vi "Remove Group.vi"(8 "error in (no error)":errorcluster, 10 "ID":string, 11 "Configuration Session in":refnum<class "Configuration Session.lvclass">) -> (0 "error out":errorcluster, 3 "Configuration Session out":refnum<class "Configuration Session.lvclass">, 4 "exists?":bool)   [LabVIEW 2017, in "DSF Core.lvlib" / "Configuration Session.lvclass"]
doc: "Removes a section from the configuration data identified by <B>dsf refnum</B>."
uses:
  Configuration Session.lvclass
  Configuration Session.lvclass/Configuration Session.ctl
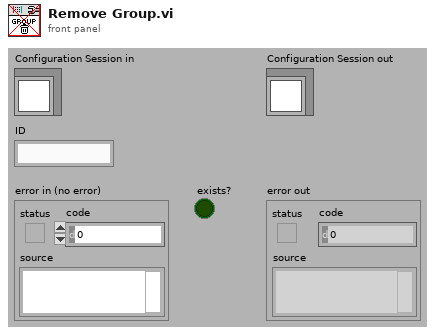
[diagram p1: front panel]
types:
  T1 = typedef "DSF Core.lvlib/Configuration Session.lvclass/DSF Config Data Ref.ctl" = refnum<data-value>
  T2 = typedef "DSF Core.lvlib/Configuration Session.lvclass/DSF Config Data.ctl" = cluster{"dsf configuration":T3, "path":path, "dirty":bool}
  T3 = typedef "DSF Core.lvlib/Configuration Session.lvclass/Internal DSF Configuration.ctl" = cluster{"dsfversion":T4, "version":T4, "plugins":T5[], "groups":T10[], "transfers":T12[], "channels":T14[], "settings":T16[], "framework configuration":T18}
  T4 = typedef "DSF Core.lvlib/DSF Version Info.ctl" = cluster{"major":u32, "minor":u32, "fix":u32, "build":string}
  T5 = typedef "DSF Core.lvlib/Configuration Session.lvclass/Internal DSF Plugin with ID.ctl" = cluster{"id":string, "values":T6}
  T6 = typedef "DSF Core.lvlib/Configuration Session.lvclass/Internal DSF Plugin Info.ctl" = cluster{"components":string[], "timing":T7, "group ids":string[], "settings id":string, "threads":T8[]}
  T7 = typedef "DSF Core.lvlib/DSF Timing Info.ctl" = cluster{"priority":u64, "decimation":u64, "offset":u64}
  T8 = typedef "DSF Core.lvlib/DSF Engine Plugin Thread Configuration.ctl" = cluster{"buffer converter settings":T9, "transceiver settings":T9, "custom settings":T9, "processor":i32, "priority offset":i16}
  T9 = typedef "DSF Core.lvlib/DSF Settings Info.ctl" = cluster{"key":string, "value":string}[]
  T10 = typedef "DSF Core.lvlib/Configuration Session.lvclass/Internal DSF Group with ID.ctl" = cluster{"id":string, "values":T11}
  T11 = typedef "DSF Core.lvlib/Configuration Session.lvclass/Internal DSF Group Info.ctl" = cluster{"direction":i32, "timing":T7, "transfer ids":string[], "settings id":string, "thread":i32, "timeout behavior":u8}
  T12 = typedef "DSF Core.lvlib/Configuration Session.lvclass/Internal DSF Transfer with ID.ctl" = cluster{"id":string, "values":T13}
  T13 = typedef "DSF Core.lvlib/Configuration Session.lvclass/Internal DSF Transfer Info.ctl" = cluster{"byte order":i32, "channel ids":string[], "settings id":string}
  T14 = typedef "DSF Core.lvlib/Configuration Session.lvclass/Internal DSF Channel with ID.ctl" = cluster{"id":string, "values":T15}
  T15 = typedef "DSF Core.lvlib/Configuration Session.lvclass/Internal DSF Channel Info.ctl" = cluster{"string buffer offset":u64, "string data type":i32, "engine data type":i32, "settings id":string, "units":string}
  T16 = typedef "DSF Core.lvlib/Configuration Session.lvclass/Internal DSF Settings with ID.ctl" = cluster{"id":string, "values":T17}
  T17 = typedef "DSF Core.lvlib/Configuration Session.lvclass/Internal DSF Settings Info.ctl" = cluster{"key":string, "value":string}[]
  T18 = typedef "DSF Core.lvlib/DSF Engine Framework Configuration.ctl" = cluster{"Plugins":T19[]}
  T19 = typedef "DSF Core.lvlib/DSF Engine Plugin Configuration.ctl" = cluster{"name":string, "components":string[], "cycle timing":T7, "threads":T8[], "Transfer Groups":T20[], "settings":T9}
  T20 = typedef "DSF Core.lvlib/DSF Engine Transfer Group Configuration.ctl" = cluster{"name":string, "direction":T21, "cycle timing":T7, "thread index":i32, "settings":T9, "Transfers":T22[], "timeout behavior":T26}
  T21 = typedef "DSF Core.lvlib/DSF Direction.ctl" = enum8{"Tx", "Rx"}
  T22 = typedef "DSF Core.lvlib/DSF Engine Transfer Configuration.ctl" = cluster{"name":string, "byte order":T23, "settings":T9, "channels":T24[]}
  T23 = typedef "DSF Core.lvlib/DSF Byte Order.ctl" = enum8{"big-endian", "little-endian"}
  T24 = typedef "DSF Core.lvlib/DSF Engine Channel Configuration.ctl" = cluster{"string offset":u64, "string data type":T25, "engine data type":T25, "name":string, "settings":T9, "units":string}
  T25 = typedef "DSF Core.lvlib/DSF Data Type.ctl" = enum8{"Bool", "SGL", "DBL", "I8", "I16", "I32", "I64", "U8", "U16", "U32", "U64"}
  T26 = typedef "DSF Core.lvlib/DSF Timeout Behavior.ctl" = enum8{"Increment Late Count", "Throw Error"}
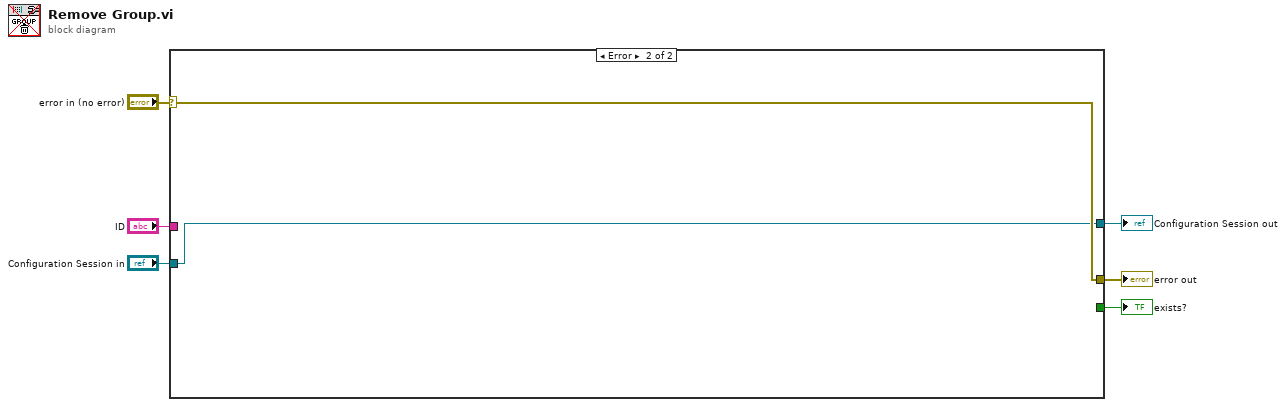
[diagram p0: block diagram]
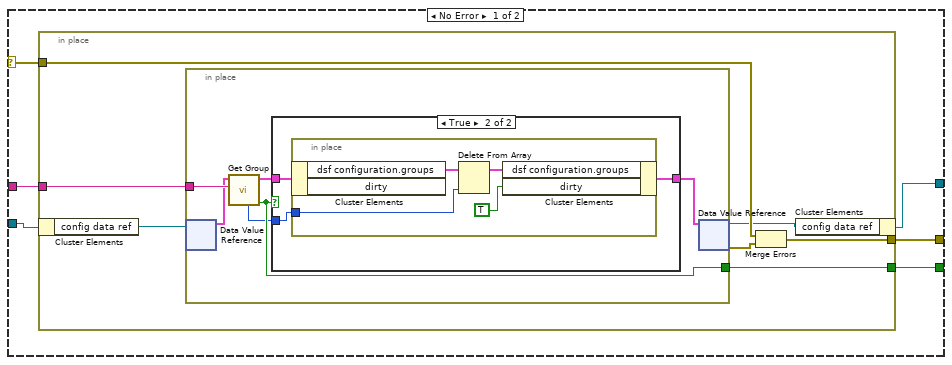
[diagram p2: hidden frame]
diagram:
  n1 = case shown="Error" "error in (no error)" {
    selector: "error in (no error)" -> [w10 w35]
    tunnel: [w9 w35] -> w2
    tunnel: [w7 w34] -> w1
    tunnel: "Configuration Session in" -> [w8 w34]
    tunnel: "ID" -> [w12 _]
    tunnel: [w11 _] -> w3
    frame No Error {
      n2 = in-place {
        in-place-border: w12 -> [w19]
        in-place-border: [w18] -> w11
        in-place-border: w10 -> [w17]
        in-place-border: [w16] -> w9
        n3 = in-place-cluster #1(w8) -> ("config data ref"=w14:T1)
        n4 = in-place {
          in-place-border: w19 -> [w25]
          in-place-border: [w24] -> w18
          n5 = in-place-dvr #2(w14) -> (w21:T2)  [unwired: 1 out]
          n6 = call "Get Group.vi"("id"=w25, "DSF Configuration in"=w21) -> ("exists?"=w24:bool, "DSF Configuration out"=w23:T2, "index"=w22:i32)  [unwired: 6 in, 1 out]
          n7 = case shown="True" w24 {
            tunnel: [w26 w29] -> w20
            tunnel: w22 -> [_ w28]
            tunnel: w23 -> [w26 w27]
            frame False {
            }
            frame True {
              n8 = in-place {
                in-place-border: w28 -> [w33]
                n9 = in-place-cluster #3(w27) -> ("dsf configuration.groups"=w32:T10[])  [unwired: 1 out]
                n10 = Delete From Array(array=w32, index=w33) -> (array with subset deleted=w31:T10[])  [unwired: 1 in, 1 out]
                n11 = in-place-cluster #3("dsf configuration.groups"=w31, "dirty"=TRUE) -> (w29:T2)
              }
            }
          }
          n12 = in-place-dvr #2(w20) -> (w13:T1, w15:errorcluster)
        }
        n13 = Merge Errors(w17, w15) -> (w16:errorcluster)
        n14 = in-place-cluster #1("config data ref"=w13) -> (w7:refnum<class "Configuration Session.lvclass">)
      }
    }
    frame Error {
    }
  }
  "error out" <- w2
  "exists?" <- w3
  "Configuration Session out" <- w1
